vi "Msg To Self.vi"(9 "Priority Msg?":bool, 10 "Msg":refnum<class "Msg Strategy.lvclass">, 11 "Actor in":refnum<class "Actor.lvclass">) -> (0 "error out":errorcluster)   [LabVIEW 2021, in "LVCAM.lvlib" / "Actor.lvclass"]
uses:
  Actor.lvclass
  Msg Strategy/Msg Strategy.lvclass
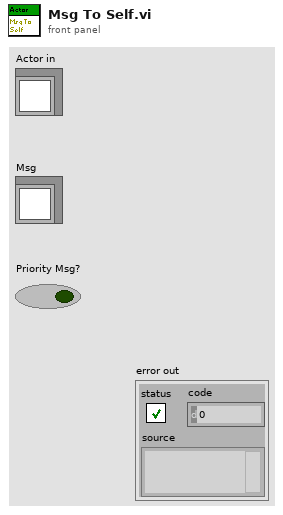
[diagram p1: front panel]
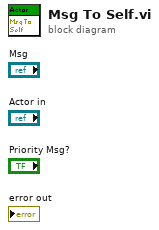
[diagram p0: block diagram]
diagram:
